vi "StandAloneViDetect.vi"(9 "call chain":string[](array[string]), 11 "VI in":refnum<vi>) -> (1 "VI Name":string, 2 "standalone(t)":bool)   [LabVIEW 2018]
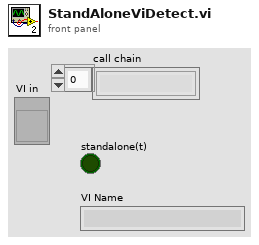
[diagram p1: front panel]
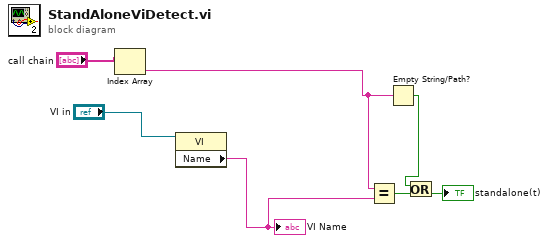
[diagram p0: block diagram]
diagram:
  n1 = Index Array(array="call chain") -> (element=w2:string)  [unwired: 1 in]
  n2 = property class="VI"(reference="VI in") -> ("Name"=w6:string)  [unwired: 1 in, 2 out]
  "VI Name" <- w6
  n3 = Equal?(x=w2, y=w6) -> (x = y?=w7:bool)
  n4 = Empty String/Path?(string/path=w2) -> (empty?=w1:bool)
  n5 = Or(x=w1, y=w7) -> (x .or. y?=→"standalone(t)":bool)
